vi "wheelS.vi"(7 "方向":dbl format="%#_13g") -> (8 "輪速比":dbl[](array[numeric]))   [LabVIEW 2019]
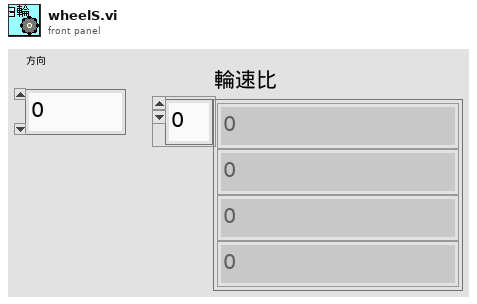
[diagram p1: front panel]
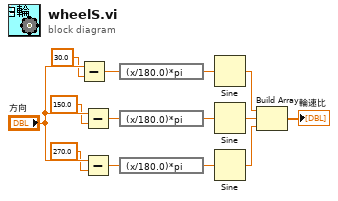
[diagram p0: block diagram]
diagram:
  n1 = Subtract(x="方向", y=30.0) -> (x-y=w14:dbl)
  n2 = Subtract(x="方向", y=150.0) -> (x-y=w12:dbl)
  n3 = Subtract(x="方向", y=270.0) -> (x-y=w13:dbl)
  n4 = expression code="(x/180.0)*pi" ("degrees to radians")(w14) -> (w9:dbl)
  n5 = expression code="(x/180.0)*pi" ("degrees to radians")(w12) -> (w11:dbl)
  n6 = expression code="(x/180.0)*pi" ("degrees to radians")(w13) -> (w8:dbl)
  n7 = Sine(x=w9) -> (sin(x)=w7:dbl)
  n8 = Sine(x=w11) -> (sin(x)=w10:dbl)
  n9 = Sine(x=w8) -> (sin(x)=w6:dbl)
  n10 = Build Array(w7, w10, w6) -> (→"輪速比":dbl[])
